vi "Support FVIR Setup.vi"(0 "UI":refnum<queue>, 1 "Modbus":refnum<queue>, 2 "Initialize?":bool, 3 "Alicat_GasMeter":refnum<queue>, 5 "Vesta FVIR":refnum<queue>, 7 "Vesta ON Temperature (FVIR)":u16=135, 9 "Select test case":i32(listbox), 11 "error in (no error)":errorcluster) -> (4 "UI Output":refnum<queue>, 8 "Test Case - FVIR":string, 15 "error out":errorcluster)   [LabVIEW 2020]
uses:
  Message Queue/Message Cluster.ctl
  Message Queue/Enqueue Message (Single).vi
  Message Queue/Message Queue.lvlib
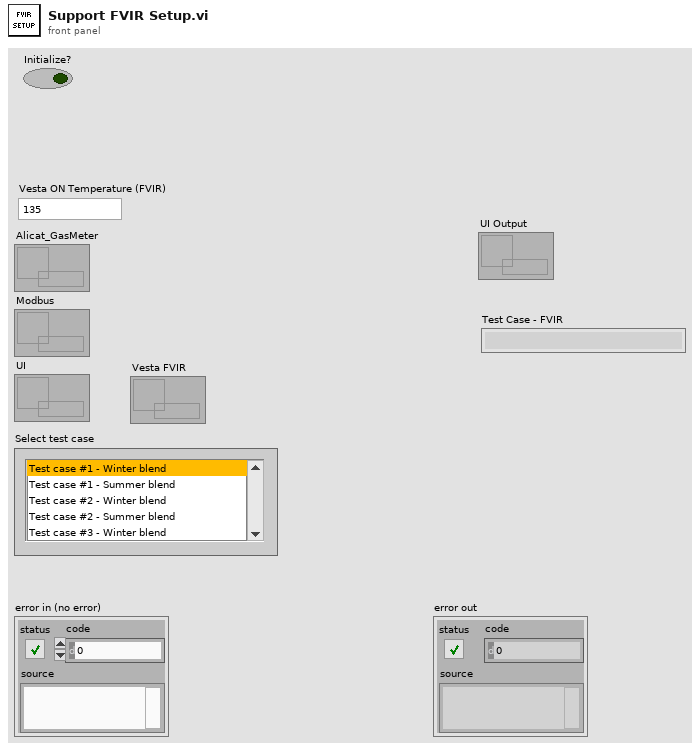
[diagram p1: front panel]
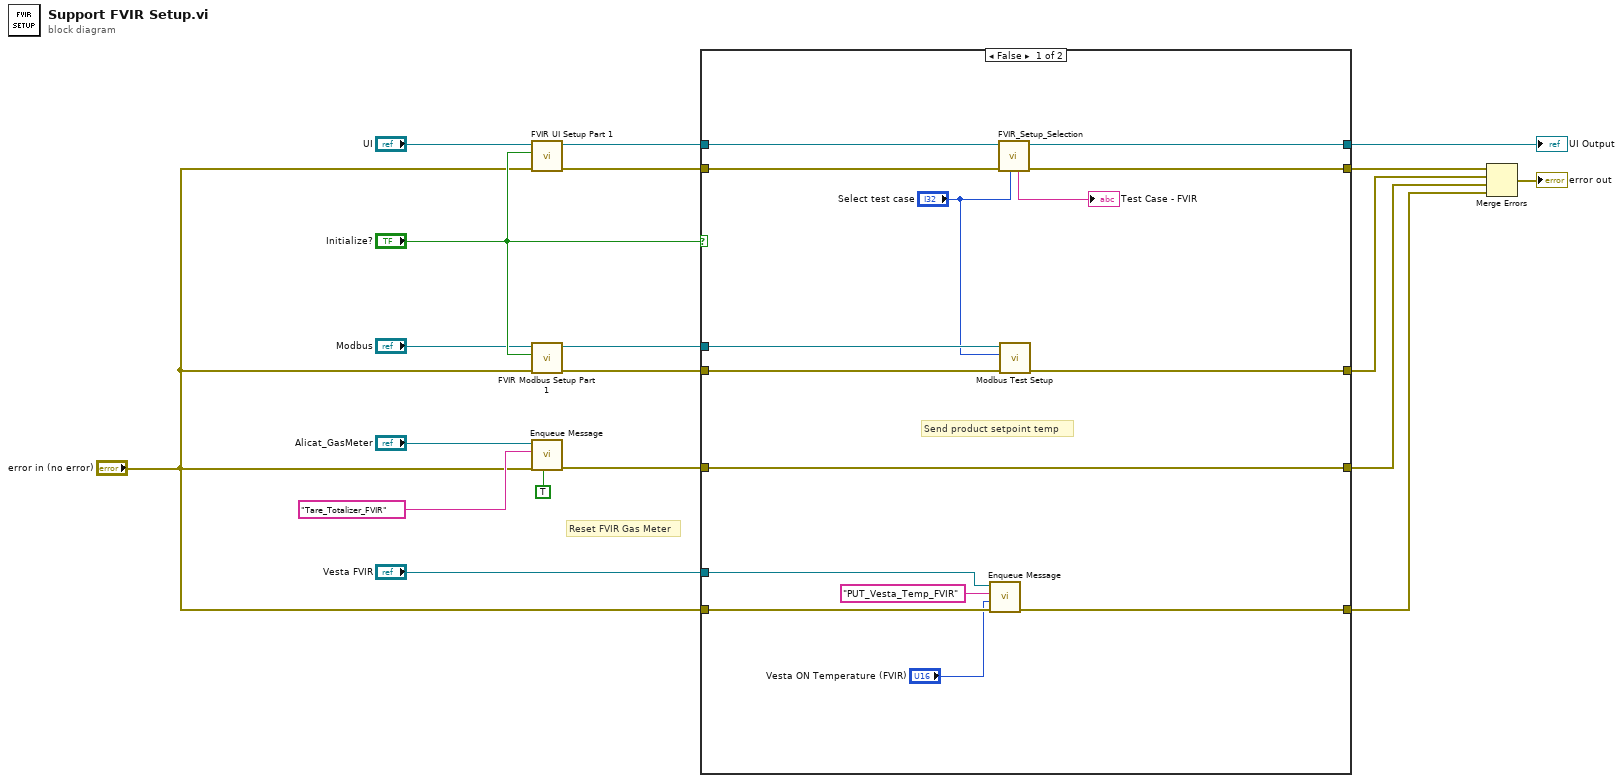
[diagram p0: block diagram]
diagram:
  # "Reset FVIR Gas Meter"
  n1 = call "FVIR UI Setup Part 1.vi"("error in (no error)"="error in (no error)", "Initialize? in"="Initialize?", "Queue in"="UI") -> ("error out"=w12:errorcluster, "Queue out"=w15:refnum<queue>)  [unwired: 7 in]
  n2 = call "FVIR Modbus Setup Part 1.vi"("error in (no error)"="error in (no error)", "Initialize? in"="Initialize?", "Queue in"="Modbus") -> ("error out"=w11:errorcluster, "Queue out"=w14:refnum<queue>)  [unwired: 7 in]
  n3 = call-poly "Enqueue Message.vi"("Priority Message? (F)"=TRUE, "error in (no error)"="error in (no error)", "Message"="Tare_Totalizer_FVIR", "Message Queue"="Alicat_GasMeter") -> ("error out"=w10:errorcluster)  [unwired: 6 in, 1 out]
  n4 = case shown="False" "Initialize?" {
    tunnel: w11 -> [w30 w39]
    tunnel: [w27 w39] -> w8
    tunnel: w14 -> [w29 _]
    tunnel: w15 -> [w34 w35]
    tunnel: w12 -> [w33 w38]
    tunnel: [w31 w38] -> w9
    tunnel: w10 -> [w26 w37]
    tunnel: [w26 w37] -> w7
    tunnel: "error in (no error)" -> [w23 w36]
    tunnel: [w22 w36] -> w6
    tunnel: [w25 w35] -> w4
    tunnel: "Vesta FVIR" -> [w20 _]
    frame False {
      # "Send product setpoint temp"
      n5 = call-poly "Enqueue Message.vi"("error in (no error)"=w23, "Message Data"="Vesta ON Temperature (FVIR)", "Message"="PUT_Vesta_Temp_FVIR", "Message Queue"=w20) -> ("error out"=w22:errorcluster)  [unwired: 6 in, 1 out]
      n6 = call "FVIR_Setup_Selection.vi"("Select test case"="Select test case", "error in (no error)"=w33, "UI in"=w34) -> ("error out"=w31:errorcluster, "UI out"=w25:refnum<queue>, "Test Case - FVIR"=→"Test Case - FVIR":string)  [unwired: 6 in]
      n7 = call "Modbus Test Setup.vi"("error in (no error)"=w30, "Select test case"="Select test case", "Queue in"=w29) -> ("error out"=w27:errorcluster)  [unwired: 7 in, 1 out]
    }
    frame True {
    }
  }
  "UI Output" <- w4
  n8 = Merge Errors(w9, w8, w7, w6) -> (→"error out":errorcluster)
